vi "FemtoGain_ReadAll.vi"(11 "Amplifier Settings":u16[](array[ring])=[0, 1, 2, 3] items=["DDPCA1", "DDPCA2", "DLPVA1", "DLPVA2"]) -> (3 "Femto Gains":i32[](array[numeric])=[1000000, 1000000, 1000, 1000])   [LabVIEW 2013]
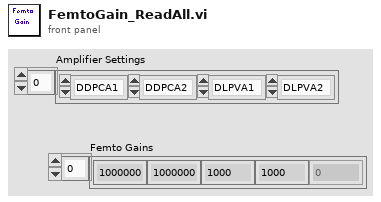
[diagram p1: front panel]
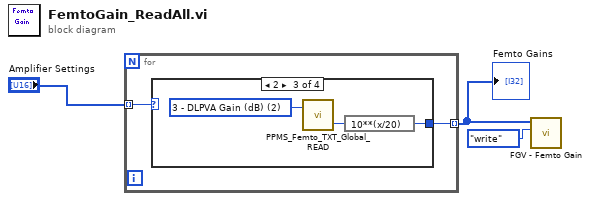
[diagram p0: block diagram]
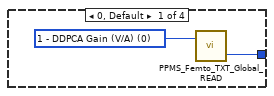
[diagram p2: hidden frame]
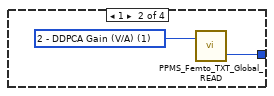
[diagram p3: hidden frame]
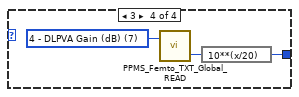
[diagram p4: hidden frame]
diagram:
  n1 = for {
    tunnel: "Amplifier Settings" -> [w5] mode=indexing
    tunnel: [w4] -> w2 mode=indexing
    n2 = case shown="2" w5 {
      tunnel: [w7 w9 w10 w13] -> w4
      frame 0, Default {
        w6 = u16 0 items=["1 - DDPCA Gain (V/A)", "2 - DDPCA Gain (V/A)", "3 - DLPVA Gain (dB)", "3 - Gain 1", "3 - Gain 2", "3 - AC/DC coupling", "3 - filter", "4 - DLPVA Gain (dB)", "4 - Gain 1", "4 - Gain 2", "4 - AC/DC coupling", "4 - filter"] ("Property")
        n3 = call "PPMS_Femto_TXT_Global_READ.vi"("Property"=w6) -> ("Value"=w7:i32)  [unwired: 1 in, 1 out]
      }
      frame 1 {
        w8 = u16 1 items=["1 - DDPCA Gain (V/A)", "2 - DDPCA Gain (V/A)", "3 - DLPVA Gain (dB)", "3 - Gain 1", "3 - Gain 2", "3 - AC/DC coupling", "3 - filter", "4 - DLPVA Gain (dB)", "4 - Gain 1", "4 - Gain 2", "4 - AC/DC coupling", "4 - filter"] ("Property")
        n4 = call "PPMS_Femto_TXT_Global_READ.vi"("Property"=w8) -> ("Value"=w9:i32)  [unwired: 1 in, 1 out]
      }
      frame 2 {
        w12 = u16 2 items=["1 - DDPCA Gain (V/A)", "2 - DDPCA Gain (V/A)", "3 - DLPVA Gain (dB)", "3 - Gain 1", "3 - Gain 2", "3 - AC/DC coupling", "3 - filter", "4 - DLPVA Gain (dB)", "4 - Gain 1", "4 - Gain 2", "4 - AC/DC coupling", "4 - filter"] ("Property")
        n5 = call "PPMS_Femto_TXT_Global_READ.vi"("Property"=w12) -> ("Value"=w11:i32)  [unwired: 1 in, 1 out]
        n6 = expression code="10**(x/20)"(w11) -> (w10:i32)
      }
      frame 3 {
        w14 = u16 7 items=["1 - DDPCA Gain (V/A)", "2 - DDPCA Gain (V/A)", "3 - DLPVA Gain (dB)", "3 - Gain 1", "3 - Gain 2", "3 - AC/DC coupling", "3 - filter", "4 - DLPVA Gain (dB)", "4 - Gain 1", "4 - Gain 2", "4 - AC/DC coupling", "4 - filter"] ("Property")
        n7 = call "PPMS_Femto_TXT_Global_READ.vi"("Property"=w14) -> ("Value"=w15:i32)  [unwired: 1 in, 1 out]
        n8 = expression code="10**(x/20)"(w15) -> (w13:i32)
      }
    }
  }
  "Femto Gains" <- w2
  n9 = call "FGV - Femto Gain.vi"("Function"=enum16{"write", "read"}."write", "Femto Gains"=w2) -> ()  [unwired: 4 in, 2 out]
